vi "Rec Move To Record N (CR).vi"(8 "error in (no error)":errorcluster, 10 "n (0)":i32, 11 "command-recordset reference":T1) -> (0 "error out":errorcluster, 3 "command-recordset reference out":T1)   [LabVIEW 2013, in "NI_Database_API_64.lvlib"]
doc: "Moves the cursor to point to record <B>n</B> in the recordset. To move the cursor to the last record, set <B>n</B> to -1. You cannot use this VI with a forward-only cursor. Wire data to the reference input to determine the polymorphic instance to use or manually select the instance."
uses:
  NI_Database_API_64.lvlib
  Command-Recordset.llb/Cmd-Rec Object Reference.ctl
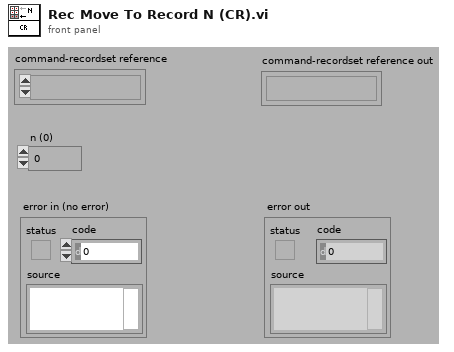
[diagram p1: front panel]
types:
  T1 = typedef "NI_Database_API_64.lvlib/Cmd-Rec Object Reference.ctl" = refnum<k1>
  T2 = typedef "NI_Database_API_64.lvlib/Cmd-Rec Data Members.ctl" = cluster{"recordset reference":T3, "command reference":T4}
  T3 = typedef "NI_Database_API_64.lvlib/Rec ObjectReference.ctl" = refnum<k1>
  T4 = typedef "NI_Database_API_64.lvlib/Cmd ObjectReference.ctl" = refnum<k1>
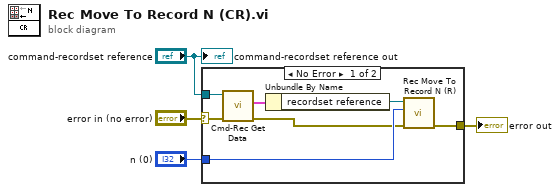
[diagram p0: block diagram]
diagram:
  n1 = case shown="No Error" "error in (no error)" {
    selector: "error in (no error)" -> [w5 w12]
    tunnel: [w11 w12] -> w4
    tunnel: "n (0)" -> [w10 _]
    tunnel: "command-recordset reference" -> [w6 _]
    frame No Error {
      n2 = call "Cmd-Rec Get Data.vi"("error in (no error)"=w5, "command-recordset reference"=w6) -> ("error out"=w8:errorcluster, "data"=w7:T2)  [unwired: 2 in, 2 out]
      n3 = Unbundle By Name(w7) -> ("recordset reference"=w9:T3)
      n4 = call "Rec Move To Record N (R).vi"("error in (no error)"=w8, "n (0)"=w10, "recordset reference"=w9) -> ("error out"=w11:errorcluster)  [unwired: 7 in, 1 out]
    }
    frame Error {
    }
  }
  "error out" <- w4
  "command-recordset reference out" <- "command-recordset reference"
